vi "Main.vi"(11 "Module Admin":refnum<class "Delacor_lib_QMH_Cloneable Module Admin.lvclass">) -> ()   [LabVIEW 2020, in "FGen.lvlib"]
doc: "This template is based off of the Queued Message Handler design pattern and the Queued Message Handler project template that ships with LabVIEW.\n\nThe main difference is that the queue is private to this module and communication between modules is performed via Broadcast and Request events.\n\nRequest events are wrapped in public API methods and are handled in the Event Handling Loop (EHL) of this VI. Any module can register for Broadcast events sent by this module. The EHL generates messages based on user interface actions.\n\nThe Message Handling Loop (MHL) processes messages generated by the EHL, or by other messages. The messages are string values, so new messages can be added easily to the Message Cases case structure in the MHL. Each message cluster can also provide an optional value for Message Data, which is a variant that can be converted to whatever message-specific data is required.\n_____\nBased on DQMH Project Template 6.0.0.91."
uses:
  FGen.lvlib
  <vilib>/Delacor/Delacor QMH/Libraries/Cloneable Module Admin_class/Delacor_lib_QMH_Cloneable Module Admin.lvclass
  C:/Program Files (x86)/National Instruments/LabVIEW 2020/vi.lib/Delacor/Delacor QMH/Libraries/Module Admin_class/Delacor_lib_QMH_Module Admin.lvclass
  Module Data--cluster.ctl
  Generador/Generador.lvclass
  <vilib>/Delacor/Delacor QMH/Libraries/Message Queue_class/Delacor_lib_QMH_Message Queue.lvclass/Delacor_lib_QMH_Message Queue.ctl
  <vilib>/Delacor/Delacor QMH/Libraries/Cloneable Module Admin_class/Delacor_lib_QMH_Cloneable Module Admin.lvclass/Delacor_lib_QMH_Cloneable Module Admin.ctl
  Stop Argument--cluster.ctl
  <vilib>/Delacor/Delacor QMH/Libraries/Module Admin_class/Delacor_lib_QMH_Module Admin.lvclass/Delacor_lib_QMH_Module Admin.ctl
  Set Signal Type Argument--cluster.ctl
  Set to Default Argument--cluster.ctl
  Generate Signal Argument--cluster.ctl
  Generate Signal (Reply Payload)--cluster.ctl
  Set Class specific Argument--cluster.ctl
  <vilib>/Utility/miscctls.llb/LVPointTypeDef.ctl
  Generador/Generador.lvclass/Generador.ctl
  <vilib>/Delacor/Delacor QMH/Libraries/Message Queue_class/Delacor_lib_QMH_Enqueue Message (Single).vi
  <vilib>/Delacor/Delacor QMH/Libraries/Cloneable Module Admin_class/Delacor_lib_QMH_Get Module ID.vi
  <vilib>/Delacor/Delacor QMH/Libraries/Module Admin_class/Delacor_lib_QMH_Get External Launch.vi
  <vilib>/Utility/error.llb/Error Cluster From Error Code.vi
  <vilib>/ErrorRing/Error Ring.xnode
  <vilib>/Delacor/Delacor QMH/Libraries/Message Queue_class/Delacor_lib_QMH_Message Queue.lvclass
panel:
  out "error out":errorcluster
  out "Status":string
  in  "Simulate EHL Error":bool
  in  "Simulate MHL Error":bool
  # "Other QMH Modules communicate with this Module via its Public API (wrappers for its Request Events).\n\nThis Module communicates with other Modules via its Broadcast Events.\nAny module that wants to get these messages, just registers for this module's Broadcast events."
  # "This template is for the Delacor Modified Queued Message Handler design pattern.\n\nSee the block diagram for more information on how to use this template."
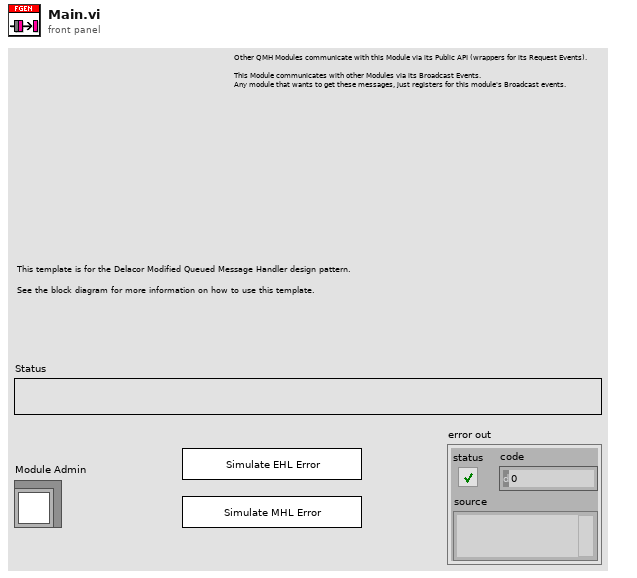
[diagram p1: front panel]
types:
  T1 = typedef "FGen.lvlib/Request Events--cluster.ctl" = cluster{"Stop Module":refnum<user-event>, "Show Panel":refnum<user-event>, "Hide Panel":refnum<user-event>, "Show Diagram":refnum<user-event>, "Get Module Execution Status":refnum<user-event>, "Set Signal Type":refnum<user-event>, "Set to Default":refnum<user-event>, "Generate Signal":refnum<user-event>, "Set Class specific":refnum<user-event>}
  T2 = typedef "FGen.lvlib/Module Data--cluster.ctl" = cluster{"Status":string, "Generator":refnum<class "Generador.lvclass">}
  T3 = enum32{"invalid lock state", "Not Locked", "Locked (No Password)", "Password-protected"}
  T4 = typedef "FGen.lvlib/Stop Argument--cluster.ctl" = cluster{"Module ID":i32, "Origin":string, "Exit via Stop Module Req?":bool, "Wait for Module to stop?":bool}
  T5 = typedef "FGen.lvlib/Set Signal Type Argument--cluster.ctl" = cluster{"Module ID":i32, "signal type":enum16{"Sine Wave", "Triangle Wave", "Square Wave", "Sawtooth Wave"}}
  T6 = typedef "FGen.lvlib/Set to Default Argument--cluster.ctl" = cluster{"Module ID":i32, "Boolean":bool}
  T7 = typedef "FGen.lvlib/Generate Signal Argument--cluster.ctl" = cluster{"Module ID":i32, "Wait Notifier":refnum<notifier>, "wait for reply":bool}
  T8 = typedef "FGen.lvlib/Set Class specific Argument--cluster.ctl" = cluster{"Module ID":i32, "Class name":string}
  T9 = typedef "LVPointTypeDef.ctl" = cluster{"Horizontal":i16, "Vertical":i16}
  T10 = enum32{"Invalid", "Standard", "Closed", "Hidden", "Minimized", "Maximized"}
  T11 = typedef "FGen.lvlib/Generate Signal (Reply Payload)--cluster.ctl" = cluster{"signal out":waveform(dbl), "Generate Signal_error":errorcluster}
  T12 = enum16{"Sine Wave", "Triangle Wave", "Square Wave", "Sawtooth Wave"}
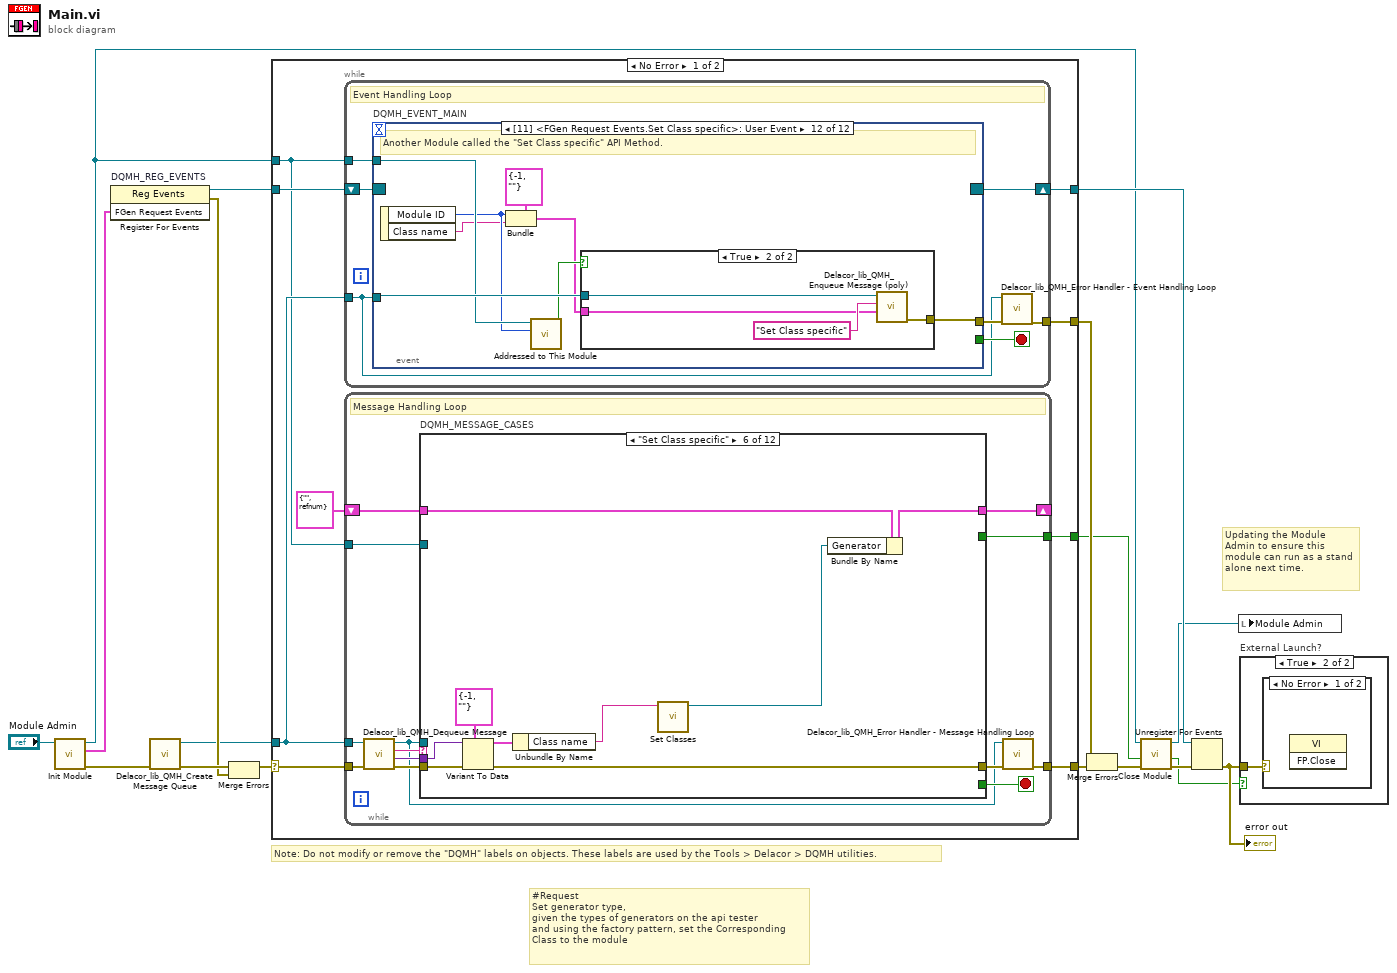
[diagram p0: block diagram]
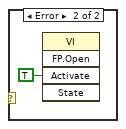
[diagram p3: hidden frame]
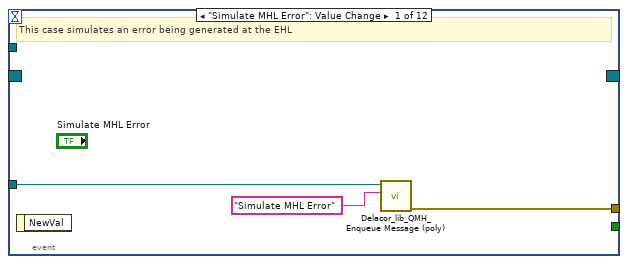
[diagram p4: hidden frame]
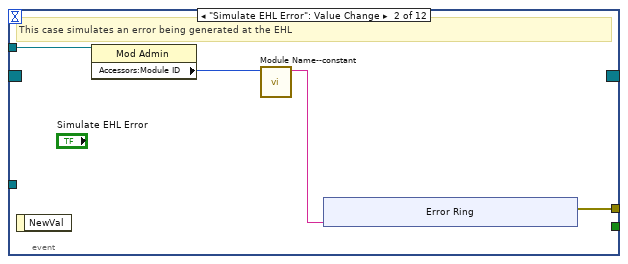
[diagram p5: hidden frame]
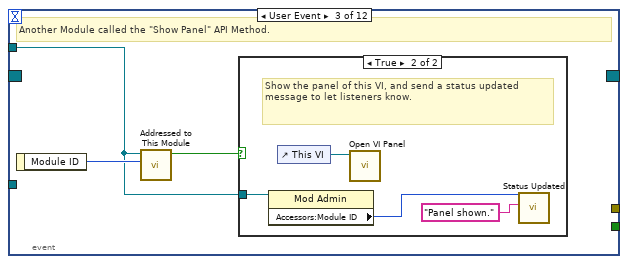
[diagram p6: hidden frame]
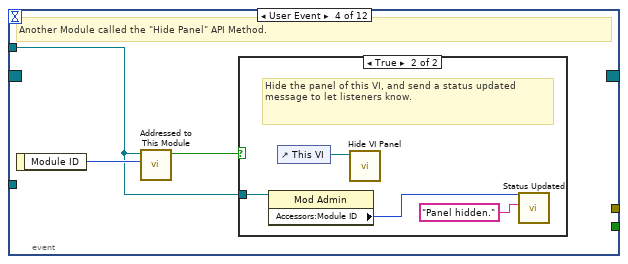
[diagram p8: hidden frame]
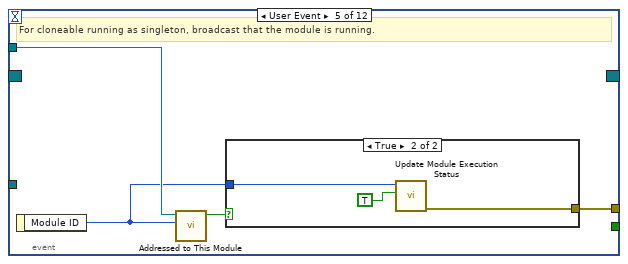
[diagram p10: hidden frame]
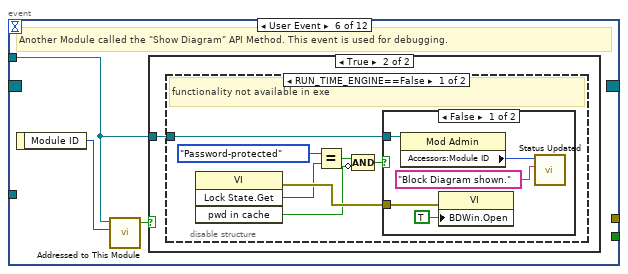
[diagram p12: hidden frame]
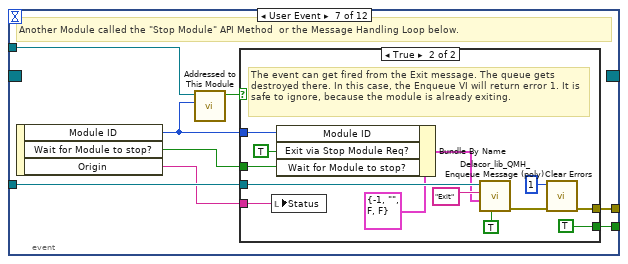
[diagram p16: hidden frame]
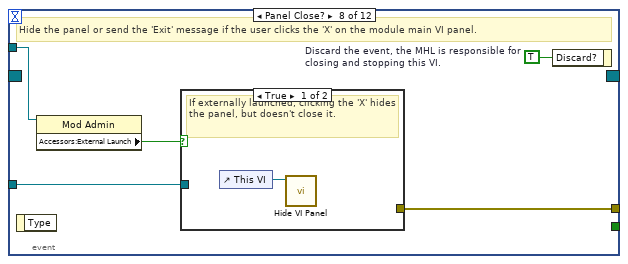
[diagram p18: hidden frame]
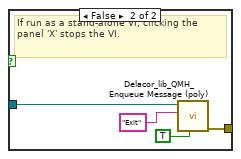
[diagram p19: hidden frame]
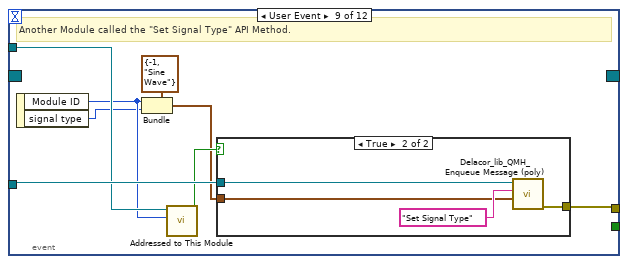
[diagram p20: hidden frame]
diagram:
  # "#Request\nSet generator type, \ngiven the types of generators on the api tester\nand using the factory pattern, set the Corresponding\nClass to the module"
  # "Note: Do not modify or remove the \"DQMH\" labels on objects. These labels are used by the Tools > Delacor > DQMH utilities."
  # "Updating the Module Admin to ensure this module can run as a stand alone next time."
  n1 = call "Init Module.vi"("Cloneable Module Admin in"="Module Admin") -> ("error out"=w15:errorcluster, "FGen Request Events"=w7:T1, "Cloneable Module Admin out"=w4:refnum<class "Delacor_lib_QMH_Cloneable Module Admin.lvclass">)  [unwired: 8 in]
  n2 = register-events "DQMH_REG_EVENTS"(w7) -> (reference out=w8:refnum<event-registration>, error out=w10:errorcluster)  [unwired: 2 in]
  n3 = call <vilib>:"Delacor_lib_QMH_Create Message Queue.vi"("error in"=w15) -> ("error out"=w12:errorcluster, "Message Queue"=w6:refnum<class "Delacor_lib_QMH_Message Queue.lvclass">)  [unwired: 9 in]
  n4 = Merge Errors(w12, w10) -> (w11:errorcluster)
  n5 = case shown="No Error" w11 {
    selector: w11 -> [w25 w317]
    tunnel: [w27 w316] -> w16
    tunnel: [w24 w324] -> w9
    tunnel: w8 -> [w22 w324]
    tunnel: w6 -> [w21 w315]
    tunnel: [w26 _] -> w17
    tunnel: w4 -> [w20 w320]
    tunnel: [w19 _] -> w2
    frame No Error {
      n6 = while {
        tunnel: w21 -> [w28]
        shift-right: [w31] -> w24
        shift-left: w22 -> [w32]
        tunnel: [w33] -> w26
        tunnel: w20 -> [w29]
        stop <- w30 stop-if-true
        # "Event Handling Loop"
        n7 = event "DQMH_EVENT_MAIN" shown="[11] <FGen Request Events.Set Class specific>: User Event" {
          selector: w32 -> [_ _ _ _ _ _ _ _ _ _ _ _]
          dyn-events: [_ _ _ _ _ _ _ _ _ _ _ _] -> w31
          timeout: _ -> [_ _ _ _ _ _ _ _ _ _ _ _]
          tunnel: [_ _ _ _ _ _ w89 _ _ _ _ _] -> w30
          tunnel: w28 -> [w36 _ _ _ _ _ w92 w108 w124 w136 w149 w161]
          tunnel: [w37 w41 _ _ w66 _ w93 w111 w117 w129 w141 w154] -> w34
          tunnel: w29 -> [_ w40 w49 w56 w64 w70 w91 w109 w122 w134 w147 w159]
          event "Simulate MHL Error": Value Change {
            # "This case simulates an error being generated at the EHL"
            n8 = event-data() -> ()  [unwired: 1 in, 1 out]
            n9 = call-poly <vilib>:"Delacor_lib_QMH_Enqueue Message (poly).vi"("Message"="Simulate MHL Error", "Message Queue in"=w36) -> ("error out"=w37:errorcluster)  [unwired: 8 in, 1 out]
          }
          event "Simulate EHL Error": Value Change {
            # "This case simulates an error being generated at the EHL"
            n10 = event-data() -> ()  [unwired: 1 in, 1 out]
            n11 = property class="Mod Admin"(reference=w40) -> ("Accessors:Module ID"=w39:i32)  [unwired: 1 in, 2 out]
            n12 = call "Module Name--constant.vi"("Module ID"=w39) -> ("Module Name"=w38:string)  [unwired: 10 in]
            n13 = xnode "Error Ring"("parameter 0"=w38) -> ("error out"=w41:errorcluster)
          }
          event User Event {
            # "Another Module called the \"Show Panel\" API Method."
            n14 = event-data() -> ("Module ID"=w50:i32)  [unwired: 1 in]
            n15 = call "Addressed to This Module.vi"("Module ID from Argument"=w50, "Module Admin"=w49) -> ("Addressed to this instance?"=w51:bool)  [unwired: 8 in, 1 out]
            n16 = case shown="True" w51 {
              tunnel: w49 -> [_ w53]
              frame False {
              }
              frame True {
                # "Show the panel of this VI, and send a status updated message to let listeners know."
                n17 = property class="Mod Admin"(reference=w53) -> ("Accessors:Module ID"=w52:i32)  [unwired: 1 in, 2 out]
                n18 = control-ref of="This VI"() -> (w55:refnum<vi>)
                n19 = call "Open VI Panel.vi"("VI"=w55) -> ()  [unwired: 10 in, 1 out]
                n20 = call "Status Updated.vi"("Status"="Panel shown." ("format string"), "Module ID"=w52) -> ()  [unwired: 9 in, 1 out]
              }
            }
          }
          event User Event {
            # "Another Module called the \"Hide Panel\" API Method."
            n21 = event-data() -> ("Module ID"=w57:i32)  [unwired: 1 in]
            n22 = call "Addressed to This Module.vi"("Module ID from Argument"=w57, "Module Admin"=w56) -> ("Addressed to this instance?"=w58:bool)  [unwired: 8 in, 1 out]
            n23 = case shown="True" w58 {
              tunnel: w56 -> [_ w60]
              frame False {
              }
              frame True {
                # "Hide the panel of this VI, and send a status updated message to let listeners know."
                n24 = property class="Mod Admin"(reference=w60) -> ("Accessors:Module ID"=w59:i32)  [unwired: 1 in, 2 out]
                n25 = control-ref of="This VI"() -> (w62:refnum<vi>)
                n26 = call "Hide VI Panel.vi"("VI"=w62) -> ()  [unwired: 10 in, 1 out]
                n27 = call "Status Updated.vi"("Status"="Panel hidden." ("format string"), "Module ID"=w59) -> ()  [unwired: 9 in, 1 out]
              }
            }
          }
          event User Event {
            # "For cloneable running as singleton, broadcast that the module is running."
            n28 = event-data() -> ("Module ID"=w63:i32)  [unwired: 1 in]
            n29 = call "Addressed to This Module.vi"("Module ID from Argument"=w63, "Module Admin"=w64) -> ("Addressed to this instance?"=w65:bool)  [unwired: 8 in, 1 out]
            n30 = case shown="True" w65 {
              tunnel: [_ w69] -> w66
              tunnel: w63 -> [_ w68]
              frame False {
              }
              frame True {
                n31 = call "Update Module Execution Status.vi"("Running?"=TRUE, "Module ID"=w68) -> ("error out"=w69:errorcluster)  [unwired: 9 in]
              }
            }
          }
          event User Event {
            # "Another Module called the \"Show Diagram\" API Method. This event is used for debugging."
            n32 = event-data() -> ("Module ID"=w71:i32)  [unwired: 1 in]
            n33 = call "Addressed to This Module.vi"("Module ID from Argument"=w71, "Module Admin"=w70) -> ("Addressed to this instance?"=w72:bool)  [unwired: 8 in, 1 out]
            n34 = case shown="True" w72 {
              tunnel: w70 -> [_ w73]
              frame False {
              }
              frame True {
                n35 = disable-structure shown="RUN_TIME_ENGINE==False" {
                  disable-tunnel: w73 -> [w74 _]
                  frame condition #0 (active) {
                    # "functionality not available in exe"
                    n36 = invoke class="VI" method="Lock State.Get"() -> (error out=w80:errorcluster, "Get Lock State"=w79:T3, "pwd in cache"=w76:bool)  [unwired: 4 in, 1 out]
                    n37 = Equal?(x=T3."Password-protected", y=w79) -> (x = y?=w77:bool)
                    n38 = Compound Arithmetic op=AND(w77, invert w76) -> (w75:bool)
                    n39 = case shown="False" w75 {
                      tunnel: w80 -> [w85 _]
                      tunnel: w74 -> [w82 _]
                      frame False {
                        n40 = property class="Mod Admin"(reference=w82) -> ("Accessors:Module ID"=w81:i32)  [unwired: 1 in, 2 out]
                        n41 = property class="VI"(error in=w85, "BDWin.Open"=TRUE ("Block Diagram Window:Open")) -> ()  [unwired: 1 in, 2 out]
                        n42 = call "Status Updated.vi"("Status"="Block Diagram shown." ("format string"), "Module ID"=w81) -> ()  [unwired: 9 in, 1 out]
                      }
                      frame True {
                        # "Password-protected VI, and the password is not in the cache. Do not show the diagram."
                      }
                    }
                  }
                  frame condition #1 {
                  }
                }
              }
            }
          }
          event User Event {
            # "Another Module called the \"Stop Module\" API Method  or the Message Handling Loop below."
            n43 = event-data() -> ("Module ID"=w87:i32, "Wait for Module to stop?"=w88:bool, "Origin"=w86:string)  [unwired: 1 in]
            n44 = call "Addressed to This Module.vi"("Module ID from Argument"=w87, "Module Admin"=w91) -> ("Addressed to this instance?"=w90:bool)  [unwired: 8 in, 1 out]
            n45 = case shown="True" w90 {
              tunnel: [_ w105] -> w93
              tunnel: w92 -> [_ w101]
              tunnel: [_ TRUE] -> w89
              tunnel: w88 -> [_ w96]
              tunnel: w87 -> [_ w98]
              tunnel: w86 -> [_ w94]
              frame False {
              }
              frame True {
                # "The event can get fired from the Exit message. The queue gets destroyed there. In this case, the Enqueue VI will return error 1. It is safe to ignore, because the module is already exiting."
                n46 = local write "Status"(w94) -> ()
                n47 = Bundle By Name(cluster=T4 {"Module ID"=-1, "Origin"="", "Exit via Stop Module Req?"=FALSE, "Wait for Module to stop?"=FALSE} ("Stop Argument"), "Module ID"=w98, "Exit via Stop Module Req?"=TRUE, "Wait for Module to stop?"=w96) -> (w95:T4)
                n48 = call-poly <vilib>:"Delacor_lib_QMH_Enqueue Message (poly).vi"("Priority Message? (F)"=TRUE, "Message Data"=w95, "Message"="Exit", "Message Queue in"=w101) -> ("error out"=w106:errorcluster)  [unwired: 6 in, 1 out]
                n49 = call <vilib>:"Clear Errors.vi"("error in (no error)"=w106, "specific error code to clear (0: all)"=1) -> ("error out"=w105:errorcluster)  [unwired: 4 in, 1 out]
              }
            }
          }
          event Panel Close? {
            w110 = TRUE  # Discard the event, the MHL is responsible for closing and stopping this VI.
            # "Hide the panel or send the 'Exit' message if the user clicks the 'X' on the module main VI panel."
            n50 = event-data() -> ()  [unwired: 1 in, 1 out]
            n51 = property class="Mod Admin"(reference=w109) -> ("Accessors:External Launch"=w107:bool)  [unwired: 1 in, 2 out]
            n52 = case shown="True" w107 {
              tunnel: w108 -> [_ w115]
              tunnel: [_ w116] -> w111
              frame True {
                # "If externally launched, clicking the 'X' hides the panel, but doesn't close it."
                n53 = control-ref of="This VI"() -> (w112:refnum<vi>)
                n54 = call "Hide VI Panel.vi"("VI"=w112) -> ()  [unwired: 10 in, 1 out]
              }
              frame False {
                # "If run as a stand-alone VI, clicking the panel 'X' stops the VI."
                n55 = call-poly <vilib>:"Delacor_lib_QMH_Enqueue Message (poly).vi"("Priority Message? (F)"=TRUE, "Message"="Exit", "Message Queue in"=w115) -> ("error out"=w116:errorcluster)  [unwired: 7 in, 1 out]
              }
            }
            n56 = event-data("Discard?"=w110) -> ()  [unwired: 1 in, 1 out]
          }
          event User Event {
            # "Another Module called the \"Set Signal Type\" API Method."
            n57 = event-data() -> ("Module ID"=w119:i32, "signal type"=w118:T12)  [unwired: 1 in]
            n58 = Bundle(cluster=T5 {"Module ID"=-1, "signal type"=enum."Sine Wave"} ("Set Signal Type Argument"), "Module ID"=w119, "signal type"=w118) -> (w120:T5)
            n59 = call "Addressed to This Module.vi"("Module ID from Argument"=w119, "Module Admin"=w122) -> ("Addressed to this instance?"=w123:bool)  [unwired: 8 in, 1 out]
            n60 = case shown="True" w123 {
              tunnel: w124 -> [_ w128]
              tunnel: w120 -> [_ w126]
              tunnel: [_ w125] -> w117
              frame False {
              }
              frame True {
                n61 = call-poly <vilib>:"Delacor_lib_QMH_Enqueue Message (poly).vi"("Message Data"=w126, "Message"="Set Signal Type", "Message Queue in"=w128) -> ("error out"=w125:errorcluster)  [unwired: 7 in, 1 out]
              }
            }
          }
          event User Event {
            # "Another Module called the \"Set to Default\" API Method."
            n62 = event-data() -> ("Module ID"=w131:i32, "Boolean"=w130:bool)  [unwired: 1 in]
            n63 = Bundle(cluster=T6 {"Module ID"=-1, "Boolean"=FALSE} ("Set to Default Argument"), "Module ID"=w131, "Boolean"=w130) -> (w132:T6)
            n64 = call "Addressed to This Module.vi"("Module ID from Argument"=w131, "Module Admin"=w134) -> ("Addressed to this instance?"=w135:bool)  [unwired: 8 in, 1 out]
            n65 = case shown="True" w135 {
              tunnel: w136 -> [_ w140]
              tunnel: w132 -> [_ w138]
              tunnel: [_ w137] -> w129
              frame False {
              }
              frame True {
                n66 = call-poly <vilib>:"Delacor_lib_QMH_Enqueue Message (poly).vi"("Message Data"=w138, "Message"="Set to Default", "Message Queue in"=w140) -> ("error out"=w137:errorcluster)  [unwired: 7 in, 1 out]
              }
            }
          }
          event User Event {
            # "Another Module called the \"Generate Signal\" API Method."
            n67 = event-data() -> ("Module ID"=w144:i32, "Wait Notifier"=w143:refnum<notifier>, "wait for reply"=w142:bool)  [unwired: 1 in]
            n68 = Bundle(cluster=T7 {"Module ID"=-1, "Wait Notifier"=refnum, "wait for reply"=FALSE} ("Generate Signal Argument"), "Module ID"=w144, "Wait Notifier"=w143, "wait for reply"=w142) -> (w145:T7)
            n69 = call "Addressed to This Module.vi"("Module ID from Argument"=w144, "Module Admin"=w147) -> ("Addressed to this instance?"=w148:bool)  [unwired: 8 in, 1 out]
            n70 = case shown="True" w148 {
              tunnel: w149 -> [_ w153]
              tunnel: w145 -> [_ w151]
              tunnel: [_ w150] -> w141
              frame False {
              }
              frame True {
                n71 = call-poly <vilib>:"Delacor_lib_QMH_Enqueue Message (poly).vi"("Message Data"=w151, "Message"="Generate Signal", "Message Queue in"=w153) -> ("error out"=w150:errorcluster)  [unwired: 7 in, 1 out]
              }
            }
          }
          event User Event {
            # "Another Module called the \"Set Class specific\" API Method."
            n72 = event-data() -> ("Module ID"=w156:i32, "Class name"=w155:string)  [unwired: 1 in]
            n73 = Bundle(cluster=T8 {"Module ID"=-1, "Class name"=""} ("Set Class specific Argument"), "Module ID"=w156, "Class name"=w155) -> (w157:T8)
            n74 = call "Addressed to This Module.vi"("Module ID from Argument"=w156, "Module Admin"=w159) -> ("Addressed to this instance?"=w160:bool)  [unwired: 8 in, 1 out]
            n75 = case shown="True" w160 {
              tunnel: w161 -> [_ w165]
              tunnel: w157 -> [_ w163]
              tunnel: [_ w162] -> w154
              frame False {
              }
              frame True {
                n76 = call-poly <vilib>:"Delacor_lib_QMH_Enqueue Message (poly).vi"("Message Data"=w163, "Message"="Set Class specific", "Message Queue in"=w165) -> ("error out"=w162:errorcluster)  [unwired: 7 in, 1 out]
              }
            }
          }
        }
        n77 = call-dynamic "Delacor_lib_QMH_Error Handler - Event Handling Loop.vi"("error in"=w34, "Message Queue in"=w28) -> ("dup error in"=w33:errorcluster)  [unwired: 8 in, 1 out]
      }
      n78 = while {
        tunnel: w21 -> [w169]
        shift-right: [w173] -> _
        shift-left: T2 {"Status"="", "Generator"=refnum} ("Data Cluster") -> [w174]
        tunnel: w25 -> [w177]
        tunnel: [w175] -> w27
        tunnel: w20 -> [w167]
        tunnel: [w166] -> w19
        stop <- w172 stop-if-true
        # "Message Handling Loop"
        n79 = call-dynamic "Delacor_lib_QMH_Dequeue Message.vi"("error in"=w177, "Message Queue in"=w169) -> ("error out"=w176:errorcluster, "Message Data"=w170:variant, "Message"=w171:string, "Message Queue out"=w168:refnum<class "Delacor_lib_QMH_Message Queue.lvclass">)  [unwired: 6 in]
        n80 = case "DQMH_MESSAGE_CASES" shown="\"Set Class specific\"" w171 {
          selector: w171 -> [_ _ _ _ _ _ _ _ _ _ _ w302]
          tunnel: w168 -> [_ _ _ _ _ _ _ _ w253 _ w292 _]
          tunnel: w176 -> [w198 w202 w212 w221 w235 w246 w249 w251 w262 w275 w298 w304]
          tunnel: [w196 w202 w211 w220 w234 w245 w248 w251 w258 w274 w295 w305] -> w178
          tunnel: w174 -> [w189 w201 w203 w214 w223 w240 w247 w250 w257 w272 w291 w303]
          tunnel: [w188 w201 w204 w213 w222 w238 w247 w250 w257 w272 w291 w303] -> w173
          tunnel: [_ _ _ _ _ _ _ _ _ _ w290 _] -> w172
          tunnel: w170 -> [_ _ w210 w219 w233 w244 _ _ w256 _ w288 _]
          tunnel: w167 -> [w184 _ _ _ _ _ _ _ w255 w270 w284 w300]
          tunnel: [_ _ _ _ _ _ _ _ _ _ w286 _] -> w166
          frame "Initialize" {
            w181 = "Initial Message" ("Initial Message")
            # "#Factory_Pattern\nCreate a factory pattern and a broadcast\nto populate the clases Generador"
            # "Initialize - Any operation that needs to be done before the module can receive messages. Synchronize Caller Events.vi will inform Start Module.vi that the module has launched and is ready to receive messages. Module Did Init.vi will broadcast that the module initialized."
            n81 = call "Synchronize Caller Events.vi"("error in (no error)"=w198, "Module Admin"=w184) -> ("error out"=w197:errorcluster, "Module Admin out"=w183:refnum<class "Delacor_lib_QMH_Cloneable Module Admin.lvclass">)  [unwired: 8 in]
            n82 = property class="Mod Admin"(reference=w183) -> ("Accessors:Module ID"=w179:i32, "Accessors:External Launch"=w185:bool)  [unwired: 1 in, 2 out]
            n83 = call "Get name classes.vi"() -> ("Classes"=w180:string[])  [unwired: 11 in]
            n84 = call "Get list name.vi"("Classes"=w180, "Module ID"=w179) -> ()  [unwired: 9 in, 1 out]
            n85 = call "Module Name--constant.vi"("Module ID"=w179) -> ("Module Name"=w193:string)  [unwired: 10 in]
            n86 = property class="VI"("Front Panel.Title"=w193) -> (reference out=w195:refnum<vi>, error out=w200:errorcluster)  [unwired: 2 in]
            n87 = Select(t=T10."Hidden" ("State"), s=w185, f=T10."Standard" ("State")) -> (s? t:f=w190:T10)
            n88 = invoke class="VI" method="FP.Open"(reference=w195, error in=w200, "State"=w190) -> (reference out=w194:refnum<vi>, error out=w199:errorcluster)  [unwired: 2 in, 3 out]
            n89 = call "Module Name--constant.vi"("Module ID"=w179) -> ("Module Name"=w186:string)  [unwired: 10 in]
            n90 = Bundle By Name(cluster=w189, "Status"=w181) -> (w188:T2)
            n91 = invoke class="VI" method="FP.Center"(reference=w194, error in=w199) -> ()  [unwired: 1 in, 3 out]
            n92 = property on="Pane" class="Pane"("Origin"=T9 {"Horizontal"=0, "Vertical"=0}) -> ()  [unwired: 2 in, 2 out]
            n93 = call "Module Did Init.vi"("error in (no error)"=w197, "Initialized?"=TRUE, "Origin"=w186, "Module ID"=w179) -> ("error out"=w196:errorcluster)  [unwired: 7 in]
            "Status" <- w181
          }
          frame "---Module Specific---" {
            # "Separator -- The following cases handle messages specific to this Module."
          }
          frame "Set Signal Type" {
            # "#CompleteMissingCode\nAdd the output Object of the method to the Module Data"
            # "Set the Signal type to be generated"
            n94 = Variant To Data(error in=w212, type=T5 {"Module ID"=-1, "signal type"=enum."Sine Wave"} ("Set Signal Type Argument"), Variant=w210) -> (data=w208:T5, error out=w211:errorcluster)
            n95 = Unbundle By Name(w208) -> ("signal type"=w206:T12)
            n96 = Unbundle By Name(w203) -> ("Generator"=w207:refnum<class "Generador.lvclass">)
            n97 = call "Set signal type.vi"("signal type"=w206, "Generator in"=w207) -> ("Generator out"=w205:refnum<class "Generador.lvclass">)  [unwired: 8 in, 1 out]
            n98 = Bundle By Name(cluster=w203, "Generator"=w205) -> (w204:T2)
          }
          frame "Set to Default" {
            # "#CompleteMissingCode\nAdd the output Object of the method to the Module Data"
            # "Set the signal to default values"
            n99 = Variant To Data(error in=w221, type=T6 {"Module ID"=-1, "Boolean"=FALSE} ("Set to Default Argument"), Variant=w219) -> (data=w217:T6, error out=w220:errorcluster)
            n100 = Unbundle By Name(w217) -> ()  [unwired: 2 out]
            n101 = Unbundle By Name(w214) -> ("Generator"=w216:refnum<class "Generador.lvclass">)
            n102 = call-dynamic "Default--constant.vi"("Generator in"=w216) -> ("Generator out"=w215:refnum<class "Generador.lvclass">)  [unwired: 9 in, 1 out]
            n103 = Bundle By Name(cluster=w214, "Generator"=w215) -> (w213:T2)
          }
          frame "Generate Signal" {
            # "#CompleteMissingCode\nAdd the class to the method"
            # "Generate the signal with the Defined values"
            n104 = Variant To Data(error in=w235, type=T7 {"Module ID"=-1, "Wait Notifier"=refnum, "wait for reply"=FALSE} ("Generate Signal Argument"), Variant=w233) -> (data=w231:T7, error out=w234:errorcluster)
            n105 = Unbundle By Name(w223) -> ("Generator"=w225:refnum<class "Generador.lvclass">)
            n106 = Unbundle By Name(w231) -> ("Wait Notifier"=w230:refnum<notifier>, "wait for reply"=w229:bool)  [unwired: 1 out]
            n107 = call "Generate Waveform.vi"("Generator in"=w225) -> ("Waveform"=w226:waveform(dbl), "Generator out"=w224:refnum<class "Generador.lvclass">)  [unwired: 8 in, 1 out]
            n108 = Bundle By Name(cluster=w223, "Generator"=w224) -> (w222:T2)
            n109 = Bundle By Name(cluster=T11 {"signal out"={"t0"=timestamp(0 s since 1904-01-01), "dt"=1.0, "Y"=[]}, "Generate Signal_error"={"status"=FALSE, "code"=0, "source"=""}} ("Generate Signal (Reply Payload)"), "signal out"=w226) -> (w228:T11)
            n110 = case shown="True" w229 {
              tunnel: w230 -> [_ w237]
              tunnel: w228 -> [_ w236]
              frame False {
              }
              frame True {
                n111 = Send Notification(notification=w236, notifier=w237) -> ()  [unwired: 1 in, 2 out]
              }
            }
          }
          frame "Set Class specific" {
            n112 = Variant To Data(error in=w246, type=T8 {"Module ID"=-1, "Class name"=""} ("Set Class specific Argument"), Variant=w244) -> (data=w242:T8, error out=w245:errorcluster)
            n113 = Unbundle By Name(w242) -> ("Class name"=w241:string)
            n114 = call "Set Classes.vi"("Class name"=w241) -> ("specific class reference"=w239:refnum<class "Generador.lvclass">)  [unwired: 10 in]
            n115 = Bundle By Name(cluster=w240, "Generator"=w239) -> (w238:T2)
          }
          frame "---Copy This Frame---" {
            # "Duplicate this frame when creating new messages.  Change this comment in the duplicated frame to describe this message."
            n116 = Merge Errors(w249) -> (w248:errorcluster)
          }
          frame "---Exit and Error Handling---" {
            # "Separator - the following cases handle errors and exit messages."
          }
          frame "Error" {
            # "Error - Check the error message data and respond accordingly. This message is sent by the \"Error Handler\" VIs at the end of each loop in this application."
            n117 = property class="Mod Admin"(reference=w255) -> ("Accessors:External Launch"=w254:bool, "Accessors:Module ID"=w252:i32)  [unwired: 1 in, 2 out]
            n118 = Variant To Data(error in=w262, type=errorcluster {"status"=FALSE, "code"=0, "source"=""} ("error constant"), Variant=w256) -> (data=w263:errorcluster, error out=w260:errorcluster)
            n119 = call "Error Reported.vi"("Error"=w263, "Module ID"=w252) -> ()  [unwired: 9 in, 1 out]
            n120 = case shown="False" w254 {
              tunnel: [w268 _] -> w259
              tunnel: w253 -> [w266 _]
              tunnel: w263 -> [w267 _]
              frame False {
                # "If the module is running standalone, then pop up an error dialog and call the \"Exit\" message."
                n121 = call <vilib>:"Simple Error Handler.vi"("error in (no error)"=w267) -> ()  [unwired: 4 in, 5 out]
                n122 = call-poly <vilib>:"Delacor_lib_QMH_Enqueue Message (poly).vi"("Priority Message? (F)"=TRUE, "Message"="Exit", "Message Queue in"=w266) -> ("error out"=w268:errorcluster)  [unwired: 7 in, 1 out]
              }
              frame True {
                # "If the module was launched externally, calling the Error Reported broadcast VI is the only action performed by the \"Error\" message. The module's caller can then process the error appropriately."
              }
            }
            n123 = Merge Errors(w260, w259) -> (w258:errorcluster)
            n124 = local write "error out"(w258) -> ()
          }
          frame "Simulate MHL Error" {
            # "Simulate an error occurring at the MHL"
            n125 = property class="Mod Admin"(reference=w270) -> ("Accessors:Module ID"=w271:i32)  [unwired: 1 in, 2 out]
            n126 = call "Module Name--constant.vi"("Module ID"=w271) -> ("Module Name"=w269:string)  [unwired: 10 in]
            n127 = xnode "Error Ring"("parameter 0"=w269) -> ("error out"=w273:errorcluster)
            n128 = Merge Errors(w275, w273) -> (w274:errorcluster)
          }
          frame "Exit" {
            w289 = 91  # 91: not all Exit messages will have an argument
            w290 = TRUE  # Stop the VI
            # "Release the message queue reference"
            # "Exit - Exit the application."
            n129 = Variant To Data(error in=w298, type=T4 {"Module ID"=-1, "Origin"="", "Exit via Stop Module Req?"=FALSE, "Wait for Module to stop?"=FALSE} ("Stop Argument"), Variant=w288) -> (data=w285:T4, error out=w293:errorcluster)
            n130 = call <vilib>:"Clear Errors.vi"("error in (no error)"=w293, "specific error code to clear (0: all)"=w289) -> ("error out"=w297:errorcluster)  [unwired: 4 in, 1 out]
            n131 = control-ref of="This VI"() -> (w283:refnum<vi>)
            n132 = call-dynamic "Delacor_lib_QMH_Release Message Queue.vi"("error in"=w297, "Message Queue"=w292) -> ("error out"=w296:errorcluster)  [unwired: 9 in]
            n133 = call "Handle Exit.vi"("Stop Argument"=w285, "Module Admin in"=w284, "VI reference"=w283) -> ("error out"=w294:errorcluster, "Wait for Stop?"=w286:bool)  [unwired: 7 in]
            n134 = Merge Errors(w296, w294) -> (w295:errorcluster)
          }
          frame Default {
            # "'Default' case only runs if there is a message that isn't defined in any of the other cases.  Output a programming error."
            n135 = property class="Mod Admin"(reference=w300) -> ("Accessors:Module ID"=w299:i32)  [unwired: 1 in, 2 out]
            n136 = call "Module Name--constant.vi"("Module ID"=w299) -> ("Module Name"=w301:string)  [unwired: 10 in]
            n137 = xnode "Error Ring"("parameter 0"=w302, "parameter 1"=w301) -> ("error out"=w306:errorcluster)
            n138 = Merge Errors(w304, w306) -> (w305:errorcluster)
          }
        }
        n139 = call-dynamic "Delacor_lib_QMH_Error Handler - Message Handling Loop.vi"("error in"=w178, "Message Queue in"=w168) -> ("dup error in"=w175:errorcluster)  [unwired: 8 in, 1 out]
      }
    }
    frame Error {
      n140 = call "Synchronize Caller Events.vi"("Module Admin"=w320) -> ("Module Admin out"=w319:refnum<class "Delacor_lib_QMH_Cloneable Module Admin.lvclass">)  [unwired: 9 in, 1 out]
      n141 = property class="Mod Admin"(reference=w319) -> ("Accessors:Module ID"=w318:i32)  [unwired: 1 in, 2 out]
      n142 = call-dynamic "Delacor_lib_QMH_Release Message Queue.vi"("error in"=w317, "Message Queue"=w315) -> ("error out"=w316:errorcluster)  [unwired: 9 in]
      n143 = call "Module Name--constant.vi"("Module ID"=w318) -> ("Module Name"=w323:string)  [unwired: 10 in]
      n144 = Format Into String(format string="An error occurred during initialization. %s is no longer running.", w323) -> (resulting string=w321:string)  [unwired: 2 in, 1 out]
      n145 = call "Error Reported.vi"("Additional Information"=w321, "Error"=w316, "Module ID"=w318) -> ()  [unwired: 8 in, 1 out]
    }
  }
  n146 = Merge Errors(w17, w16) -> (w18:errorcluster)
  n147 = call "Close Module.vi"("error in"=w18, "Wait for stop?"=w2, "Module Admin in"=w4) -> ("error out"=w14:errorcluster, "External Launch"=w1:bool, "Module Admin out"=w3:refnum<class "Delacor_lib_QMH_Cloneable Module Admin.lvclass">)  [unwired: 6 in]
  n148 = Unregister For Events(event registration refnum=w9, error in=w14) -> (error out=w13:errorcluster)
  "error out" <- w13
  n149 = local write "Module Admin"(w3) -> ()
  n150 = case "External Launch?" shown="True" w1 {
    tunnel: w13 -> [_ w325]
    frame False {
    }
    frame True {
      n151 = case shown="No Error" w325 {
        frame No Error {
          n152 = invoke class="VI" method="FP.Close"() -> ()  [unwired: 3 in, 3 out]
        }
        frame Error {
          n153 = invoke class="VI" method="FP.Open"("Activate"=TRUE ("Activate?")) -> ()  [unwired: 4 in, 5 out]
        }
      }
    }
  }
